vi "Or77200_ReadPos.vi"(8 "error In":errorcluster caption="error out", 11 "Port":refnum<visa-resource-name>) -> (0 "sortie d'erreur":errorcluster, 2 "Lambda Out (nm)":dbl, 3 "Port Out":refnum<visa-resource-name>)   [LabVIEW 2010]
uses:
  <vilib>/Utility/config.llb/Read Key (Double).vi
  <vilib>/Utility/config.llb/NI_LVConfig.lvlib
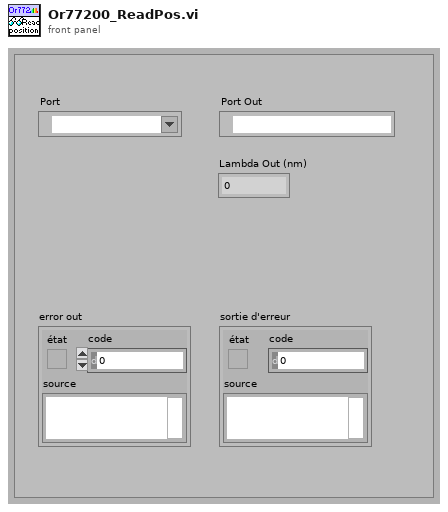
[diagram p1: front panel]
types:
  T1 = typedef "NI_LVConfig.lvlib/Config Data RefNum.ctl" = refnum<k1>
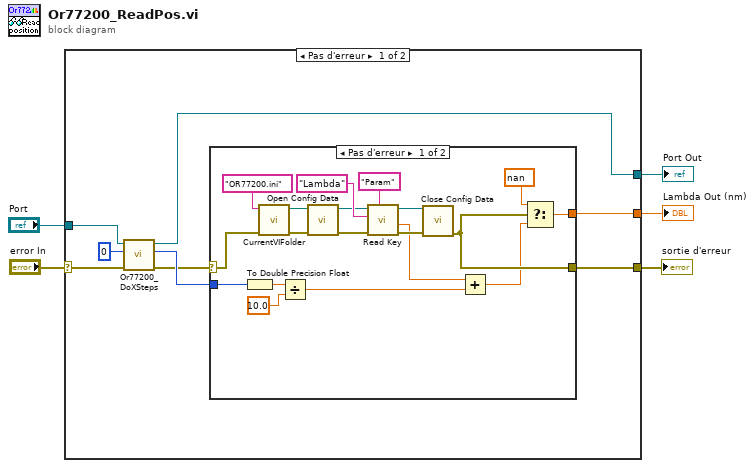
[diagram p0: block diagram]
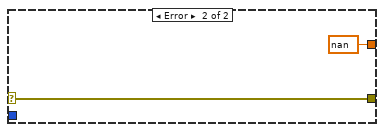
[diagram p2: hidden frame]
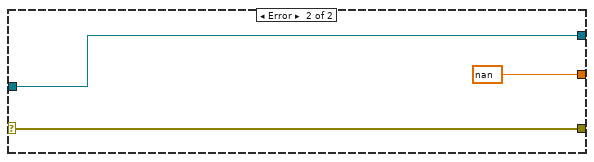
[diagram p3: hidden frame]
diagram:
  n1 = case shown="Pas d'erreur" "error In" {
    selector: "error In" -> [w11 w36]
    tunnel: "Port" -> [w13 w37]
    tunnel: [w7 w36] -> w4
    tunnel: [w6 w37] -> w3
    tunnel: [w8 nan ("cas vrai")] -> w1
    frame No Error {
      n2 = call <userlib>:"Or77200_DoXSteps.vi"("error In"=w11, "Steps"=u32 0, "Port"=w13) -> ("sortie d'erreur"=w9:errorcluster, "sortie 1"=w10:i32, "Port Out"=w6:refnum<visa-resource-name>)  [unwired: 6 in]
      n3 = case shown="Pas d'erreur" w9 {
        selector: w9 -> [w18 w33]
        tunnel: w10 -> [w30 _]
        tunnel: [w15 nan] -> w8
        tunnel: [w17 w33] -> w7
        frame No Error {
          n4 = To Double Precision Float(number=w30) -> (double precision float=w32:dbl)
          n5 = call <userlib>:"CurrentVIFolder.vi"("error in (no error)"=w18, "NomFichier"="OR77200.ini") -> ("error out"=w22:errorcluster, "Chemin"=w21:path)  [unwired: 7 in, 1 out]
          n6 = Divide(x=w32, y=10.0) -> (x/y=w20:dbl)
          n7 = call <vilib>:"Open Config Data.vi"("error in (no error)"=w22, "configuration file path"=w21) -> ("error out"=w23:errorcluster, "refnum"=w24:T1)  [unwired: 7 in, 1 out]
          n8 = call-poly <vilib>:"Read Key.vi"("section"="Param", "error in (no error)"=w23, "key"="Lambda", "refnum"=w24) -> ("error out"=w27:errorcluster, "value"=w19:dbl, "refnum out"=w28:T1)  [unwired: 4 in, 1 out]
          n9 = call <vilib>:"Close Config Data.vi"("error in (no error)"=w27, "refnum"=w28) -> ("error out"=w17:errorcluster)  [unwired: 8 in, 1 out]
          n10 = Add(x=w19, y=w20) -> (x+y=w14:dbl)
          n11 = Select(t=nan ("cas vrai"), s=w17, f=w14) -> (s? t:f=w15:dbl)
        }
        frame Error {
        }
      }
    }
    frame Error {
    }
  }
  "sortie d'erreur" <- w4
  "Port Out" <- w3
  "Lambda Out (nm)" <- w1
